vi "TestStepsGui.vi"() -> ()   [LabVIEW 2016]
uses:
  TestStepsGui.Action.ctl
  <vilib>/Utility/miscctls.llb/LVRowAndColumnUnsignedTypeDef.ctl
  <vilib>/Utility/miscctls.llb/LVRowAndColumnTypeDef.ctl
  tools/CitTemplate/citTemplate.errData.ctl
  tools/EventLog/EventLog.EventSource.ctl
  Sequence/Sequence.Data.ctl
  Sequence/Sequence.State.ctl
  Sequence/Sequence.Step.Status.ctl
  Sequence/Sequence.Test.BreakReason.ctl
  Sequence/Sequence.Test.BreakSource.ctl
  Sequence/Sequence.Test.Status.ctl
  Sequence/Sequence.Slot.StatusData.ctl
  Sequence/Sequence.Test.Unload.Status.ctl
  Sequence/Sequence.Prod.StatusData.ctl
  Sequence/Sequence.UserActions.ctl
  Sequence/Sequence.UserData.ctl
  Sequence/Sequence.MainMode.ctl
  MainGui.TestOptions.ctl
  Sequence/Sequence.Code.Sets.ctl
  Sequence/Sequence.PlateType.ctl
  Logger/Logger.Variant.Sets.ctl
  Station/Station.Changeover.State.vi
  Station/Station.Plate.Properties.ctl
  Sequence/Sequence.Code.SerialFormat.ctl
  Drivers/V7310/LowLevel/V7310.Job.Sets.ctl
  Sequence/Sequence.Counters.ctl
  Sequence/Sequence.Global.vi
  Global/ApplicationGlobal.vi
panel:
  out "Part":string
  out "Prog":bool
  out "ClientPlate":picture
  out "Total":u16 caption="Wymagane"
  out "NOK":u16
  out "OK":u16
  out "Done":u16 caption="Zrobione"
  out "Image B":picture caption="B - 0 - ERROR - 0 %"
  out "Image A":picture caption="A - 0 - ERROR - 0 %"
  out "_loop":i32(ring)=4
  out "Started":bool
  out "Panel":refnum<vi>
  in  "StartHere...":bool
  in  "LastCodes":i32(listbox) caption="Last A"
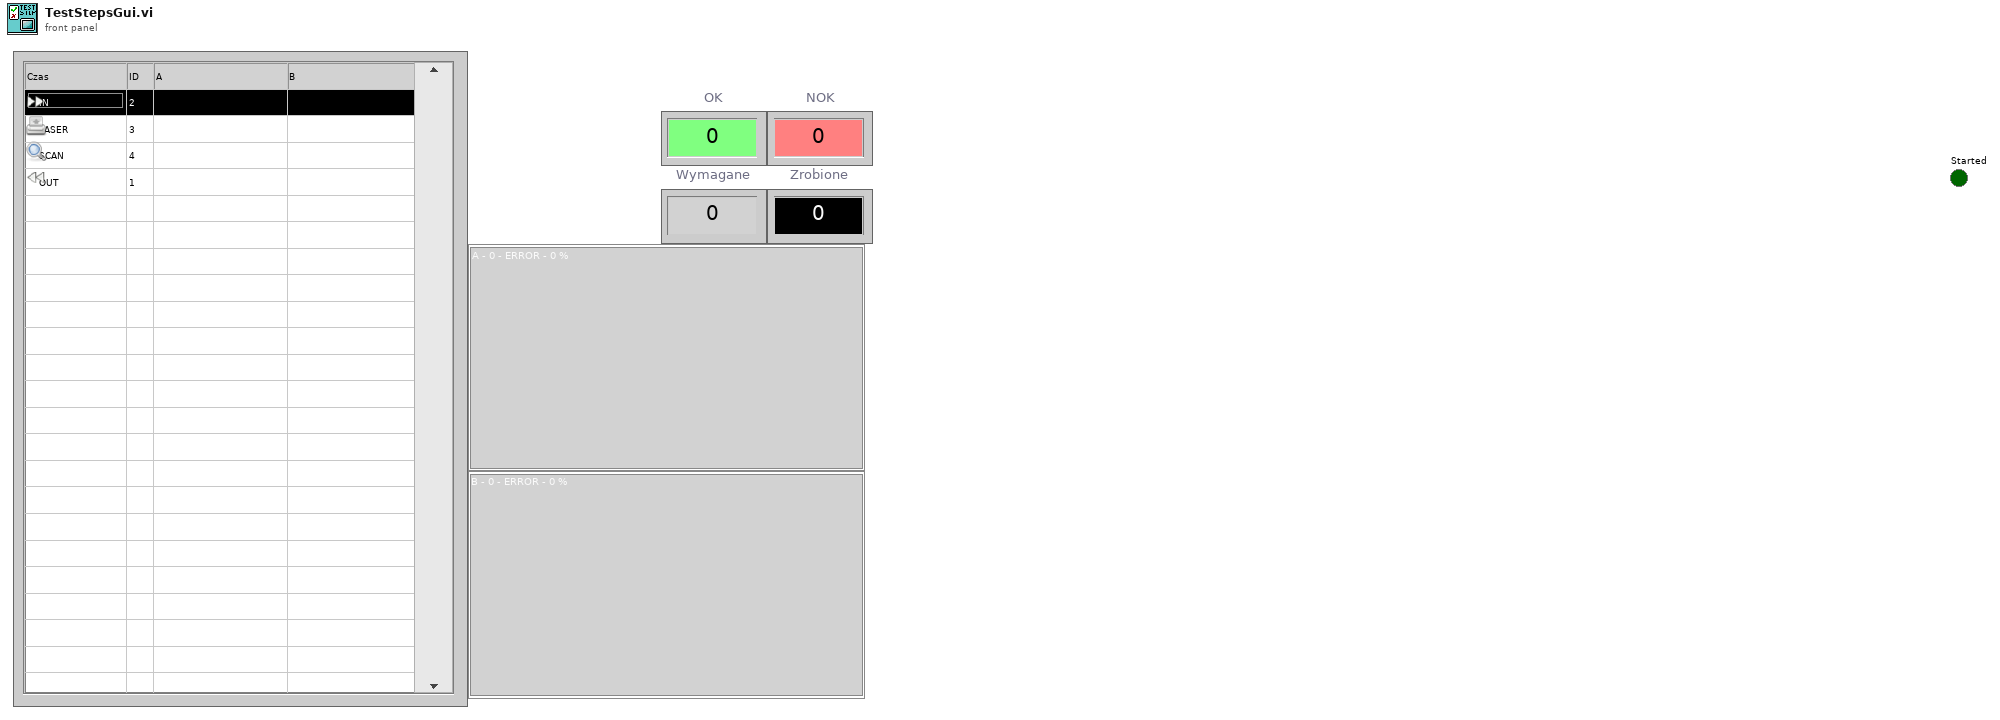
[diagram p1: front panel]
types:
  T1 = typedef "TestStepsGui.Action.ctl" = enum32{"idle", "constructor", "destructor", "--- TestStepsGui ---", "Select", "Load", "Start", "Update", "Update Images"}
  T2 = typedef "LVRowAndColumnTypeDef.ctl" = cluster{"Row":i32, "Column":i32}
  T3 = typedef "LVRowAndColumnUnsignedTypeDef.ctl" = cluster{"Row":u32, "Column":u32}
  T4 = typedef "citTemplate.errData.ctl" = cluster{"ts":timestamp, "src":T5, "instance":i32, "action":string, "error":errorcluster, "unconfirmed":bool}
  T5 = typedef "EventLog.EventSource.ctl" = enum16{"All", "Gui", "Ref", "File", "Arch", "Seq", "CPX", "DB", "Laser", "Scan.P", "Scan.O"}
  T6 = typedef "Sequence.Data.ctl" = cluster{"BeginTS":timestamp, "EndTS":timestamp, "State":T7, "Status.Work":T8, "Status.Process":T8, "Status.Home":T8, "Status.Wabco":T8, "Status.Client":T8, "BreakReason":T9, "BreakSource":T10, "DoorLock":bool, "Status.Prod":T11[], "UserAction":T15, "UserData":T16, "Error":errorcluster, "Code":T19, "Rotations":i32, "ProdIdx":i32, "ProdDone":T11[], "PrintedSerials-Wabco":i32[], "PrintedSerials-Client":i32[], "Counters-Wabco":T26, "Counters-Client":T26}
  T7 = typedef "Sequence.State.ctl" = enum16{"Init", "Idle", "Home", "Work", "Run", "Pause"}
  T8 = typedef "Sequence.Step.Status.ctl" = enum16{"-", "Pending", "Running", "Skipped", "Passed", "Failed", "Done", "Error", "Aborted", "Stopped"}
  T9 = typedef "Sequence.Test.BreakReason.ctl" = enum16{"-", "NOK container", "OK container", "Rev empty", "Rev missing", "Rev wrong", "Fork missing", "Fork wrong", "NOK limit", "Unload failure", "Single slot", "Part done", "Err: Prod move work", "Err: Prod move home", "Err: Prod lift work", "Err: Prod lift home", "Err: Prod Arm Work", "Err: Prod Arm NOK", "Err: Prod Arm OK", "Err: Prod NOK suck", "Err: Prod NOK drop", "Err: Prod OK missing", "Err: Prod OK suck", "Err: Prod OK drop"}
  T10 = typedef "Sequence.Test.BreakSource.ctl" = enum16{"-", "A", "B", "A/B"}
  T11 = typedef "Sequence.Test.Status.ctl" = cluster{"Slot":T12, "A":T14, "B":T14}
  T12 = typedef "Sequence.Slot.StatusData.ctl" = cluster{"ID":i32, "Unload":T13, "TS":timestamp, "duration":u32}
  T13 = typedef "Sequence.Test.Unload.Status.ctl" = enum16{"init", "check NOK", "check OK", "wait on NOK", "wait on OK", "wait on Unload", "done"}
  T14 = typedef "Sequence.Prod.StatusData.ctl" = cluster{"status":T8, "pause":T9, "present":bool, "printed":bool, "scanned":bool, "tuned":bool, "removed":bool, "serial":i32, "code":string, "path":path, "corners":cluster{"X":i32, "Y":i32}[], "verification":u8}
  T15 = typedef "Sequence.UserActions.ctl" = cluster{"Stop":bool, "Pause":bool, "Next":bool}
  T16 = typedef "Sequence.UserData.ctl" = cluster{"GuiMode":T17, "Test":T18, "ContinueOrder":bool}
  T17 = typedef "Sequence.MainMode.ctl" = enum16{"Process", "Base", "Order", "Manual", "Logs", "Results", "Stats", "DMC Config"}
  T18 = typedef "MainGui.TestOptions.ctl" = cluster{"IgnoreResults":bool, "IgnoreImages":bool, "ServiceMode":bool}
  T19 = typedef "Sequence.Code.Sets.ctl" = cluster{"Ready":bool, "DoubleOrder":bool, "OrderDone":bool, "AllowSingleSlot":bool, "TunedA":bool, "TunedB":bool, "CheckDM":bool, "ThresholdA":u8, "ThresholdB":u8, "Plate":T20, "ImgPath":path, "Variant":T21}
  T20 = typedef "Sequence.PlateType.ctl" = enum16{"Wabco", "Client"}
  T21 = typedef "Logger.Variant.Sets.ctl" = cluster{"State":T22, "ImgPath":path, "WabcoPlate":string, "WabcoProduct":string, "ClientProduct":string, "ClientPlate":string, "TotalQuantity":u16, "OrderQuantity":u16, "Serial":i32, "Wabco":T23, "Client":T23}
  T22 = typedef "Station.Changeover.State.vi" = enum16{"Init", "Scaning", "NOK", "Wait for ack", "Ready"}
  T23 = typedef "Station.Plate.Properties.ctl" = cluster{"LaserJob":string, "AdditionalTxt":string, "FactoryCode":string, "RevID":u8, "ForkID":u8, "FailuresLimit":u16, "GlobalCnt":i32, "Bank":u8, "SerialFormat":T24, "CoordA":T25, "CoordB":T25, "DMCconfig":i32}
  T24 = typedef "Sequence.Code.SerialFormat.ctl" = enum8{"", "6 dig", "7 dig"}
  T25 = typedef "V7310.Job.Sets.ctl" = cluster{"X":dbl, "Y":dbl, "Angle":dbl}
  T26 = typedef "Sequence.Counters.ctl" = cluster{"Expected":u16, "Done":u16, "OK":u16, "NOK":u16, "NOKlimit":u16, "Part":u16, "PartOK":u16}
  T27 = typedef "citTemplate.notifierHandle.ctl" = refnum<notifier>
  T28 = enum32{"Invalid", "Standard", "Closed", "Hidden", "Minimized", "Maximized"}
  T29 = typedef "LVPositionTypeDef.ctl" = cluster{"Left":i32, "Top":i32}
  T30 = typedef "imagedata.ctl" = cluster{"image type":i32, "image depth":i32, "image":u8[], "mask":u8[], "colors":u32[], "Rectangle":cluster{"left":i16, "top":i16, "right":i16, "bottom":i16}}
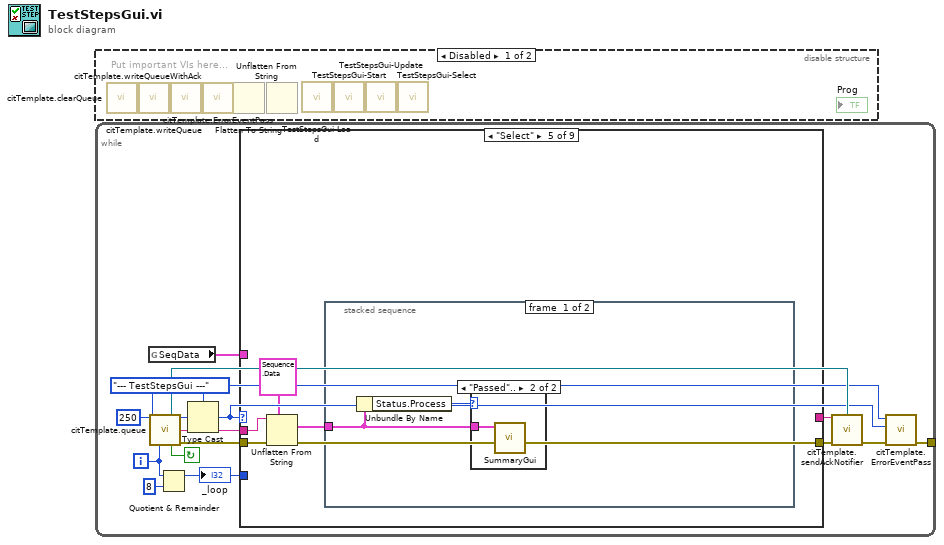
[diagram p0: block diagram]
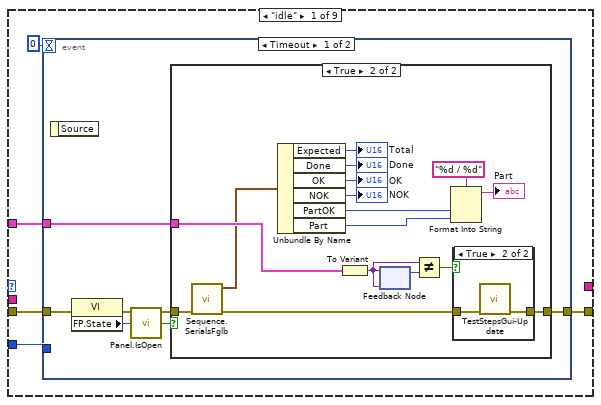
[diagram p3: hidden frame]
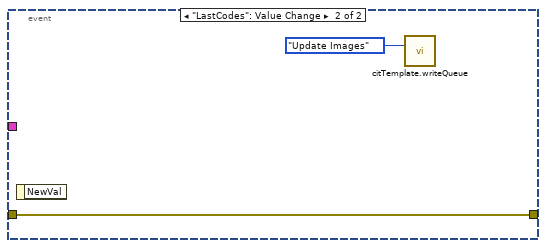
[diagram p6: hidden frame]
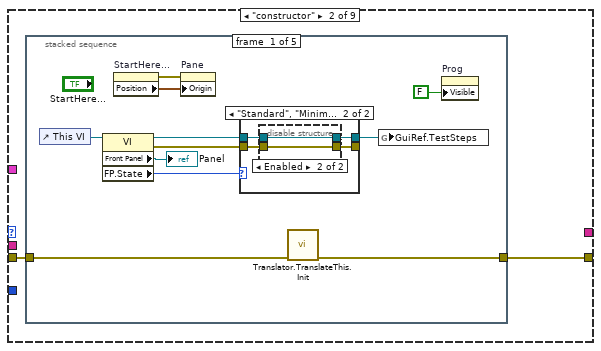
[diagram p7: hidden frame]
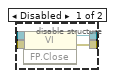
[diagram p9: hidden frame]
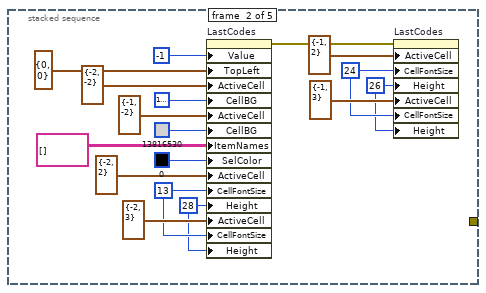
[diagram p10: hidden frame]
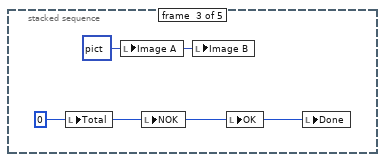
[diagram p11: hidden frame]
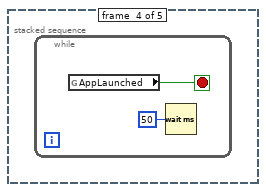
[diagram p12: hidden frame]
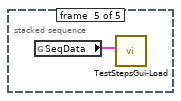
[diagram p13: hidden frame]
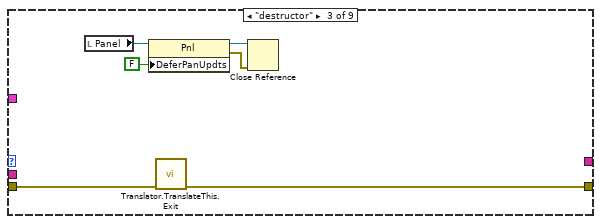
[diagram p14: hidden frame]
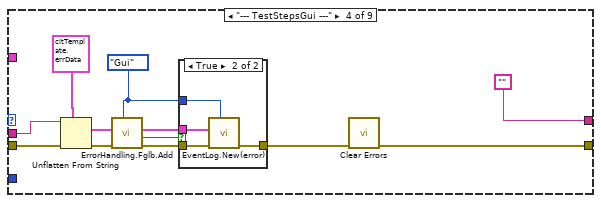
[diagram p15: hidden frame]
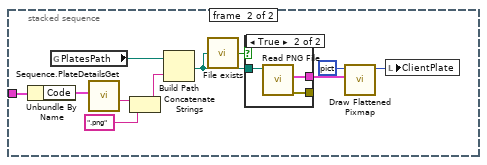
[diagram p18: hidden frame]
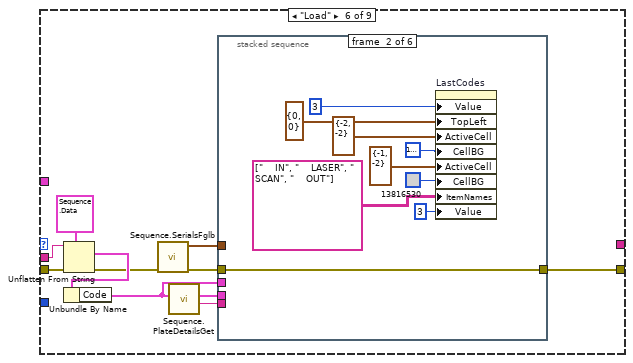
[diagram p20: hidden frame]
diagram:
  n1 = disable-structure shown="Disabled" {
    frame Disabled {
      # "Put important VIs here..."
      n2 = call "citTemplate.clearQueue.vi"() -> ()  [unwired: 14 in, 2 out]
      n3 = call "citTemplate.writeQueue.vi"() -> ()  [unwired: 15 in, 1 out]
      n4 = call "citTemplate.writeQueueWithAck.vi"() -> ()  [unwired: 13 in, 3 out]
      n5 = call "citTemplate.ErrorEventPass.vi"() -> ()  [unwired: 11 in, 1 out]
      n6 = Flatten To String() -> ()  [unwired: 4 in, 3 out]
      n7 = Unflatten From String() -> ()  [unwired: 5 in, 3 out]
      n8 = call "TestStepsGui-Load.vi"() -> ()  [unwired: 11 in, 1 out]
      n9 = call "TestStepsGui-Start.vi"() -> ()  [unwired: 11 in, 1 out]
      n10 = call "TestStepsGui-Update.vi"() -> ()  [unwired: 11 in, 1 out]
      n11 = call "TestStepsGui-Select.vi"() -> ()  [unwired: 11 in, 1 out]
    }
    frame Enabled {
    }
  }
  n12 = while {
    tunnel: [w4] -> _
    i -> [w6]
    stop <- w12 continue-if-true
    w9 = TestStepsGui.Action."--- TestStepsGui ---" ("Action")
    n13 = global read "Sequence.Global.vi" "SeqData"() -> (w1:T6)
    n14 = call "citTemplate.queue.vi"("ms timeout (250 ms)"=250, "event enum"=w9, "iteration (-1)"=w6) -> ("notifierHandle out"=w11:T27, "event out"=w15:u32, "(flatten) data out"=w14:string, "continue"=w12:bool, "error out"=w13:errorcluster)  [unwired: 2 in, 6 out]
    n15 = Quotient & Remainder(x=w6, y=8) -> (x-y*floor(x/y)=w2:i32)  [unwired: 1 out]
    "_loop" <- w2
    n16 = Type Cast(type=w9, x=w15) -> (*(type *) &x=w5:T1)
    n17 = case shown="\"Select\"" w5 {
      tunnel: w14 -> [_ _ _ w111 w121 w148 w204 _ _]
      tunnel: w13 -> [w19 w50 w100 w110 w122 w150 w205 w207 w267]
      tunnel: [_ _ _ "" _ _ _ _ _] -> w10
      tunnel: [w18 w49 w101 w103 w120 w149 w199 w208 w267] -> w8
      tunnel: w2 -> [w17 _ _ _ _ _ _ _ _]
      tunnel: w1 -> [w16 _ _ _ _ _ _ w206 w259]
      frame "idle" {
        n18 = event shown="[0] Timeout" {
          selector: _ -> [_ _]
          dyn-events: _ -> [_ _]
          timeout: 0 -> [_ _]
          tunnel: w19 -> [w26 w48]
          tunnel: [w25 w48] -> w18
          tunnel: w17 -> [_ _]
          tunnel: w16 -> [w23 _]
          event Timeout {
            n19 = event-data() -> ()  [unwired: 1 in, 1 out]
            n20 = property class="VI"(error in=w26) -> (error out=w24:errorcluster, "FP.State"=w22:T28)  [unwired: 1 in, 1 out]
            n21 = call "Panel.IsOpen.vi"("FP State"=w22) -> ("Open?"=w21:bool)
            n22 = case shown="True" w21 {
              tunnel: w24 -> [w27 w34]
              tunnel: [w27 w43] -> w25
              tunnel: w23 -> [_ w35]
              frame False {
              }
              frame True {
                n23 = call "Sequence.SerialsFglb.vi"("error in"=w34) -> ("error out"=w33:errorcluster, "Counters out"=w29:T26)  [unwired: 6 in, 3 out]
                n24 = Unbundle By Name(w29) -> ("Expected"=→"Total":u16, "Done"=→"Done":u16, "OK"=→"OK":u16, "NOK"=→"NOK":u16, "PartOK"=w32:u16, "Part"=w28:u16)
                n25 = To Variant(anything=w35) -> (Variant=w41:variant)
                n26 = feedback #1(w41) -> (w42:variant)
                n27 = feedback-in #1(w41) -> ()
                n28 = Not Equal?(x=w41, y=w42) -> (x != y?=w36:bool)
                n29 = Format Into String(format string="%d / %d", w32, w28) -> (resulting string=→"Part":string)  [unwired: 2 in, 1 out]
                n30 = case shown="True" w36 {
                  tunnel: w33 -> [w44 w45]
                  tunnel: [w44 w46] -> w43
                  frame False {
                  }
                  frame True {
                    n31 = call "TestStepsGui-Update.vi"("error in"=w45) -> ("error out"=w46:errorcluster)  [unwired: 10 in]
                  }
                }
              }
            }
          }
          event "LastCodes": Value Change {
            n32 = event-data() -> ()  [unwired: 1 in, 1 out]
            n33 = call "citTemplate.writeQueue.vi"("event in (if not connected:all statemachine with data event)"=TestStepsGui.Action."Update Images" ("Action")) -> ()  [unwired: 14 in, 1 out]
          }
        }
      }
      frame "constructor" {
        n34 = stacked-sequence {
          tunnel: w50 -> [w57 _ _ _ _]
          tunnel: [w52 _ _ _ _] -> w49
          frame #0 {
            n35 = control-ref of="This VI"() -> (w58:refnum<vi>)
            n36 = property class="VI"(reference=w58) -> (reference out=w56:refnum<vi>, error out=w55:errorcluster, "Front Panel"=→"Panel":refnum<vi>, "FP.State"=w54:T28)  [unwired: 1 in]
            n37 = property on="StartHere..." class="Bool (strict)"() -> (error out=w60:errorcluster, "Position"=w59:T29)  [unwired: 2 in, 1 out]
            n38 = property on="Pane" class="Pane"(error in=w60, "Origin"=w59) -> ()  [unwired: 1 in, 2 out]
            n39 = case shown="\"Standard\", \"Minimized\", \"Maximized\"" w54 {
              tunnel: w56 -> [w63 w67]
              tunnel: w55 -> [w62 w66]
              tunnel: [w63 w65] -> w53
              tunnel: [w62 w64] -> _
              frame Default {
              }
              frame "Standard", "Minimized", "Maximized" {
                n40 = disable-structure shown="Enabled" {
                  disable-tunnel: w67 -> [w71 w73]
                  disable-tunnel: w66 -> [w70 w72]
                  disable-tunnel: [w69 w73] -> w65
                  disable-tunnel: [w68 w72] -> w64
                  frame Disabled {
                    n41 = invoke class="VI" method="FP.Close"(reference=w71, error in=w70) -> (reference out=w69:refnum<vi>, error out=w68:errorcluster)  [unwired: 1 in, 1 out]
                  }
                  frame Enabled {
                  }
                }
              }
            }
            n42 = call "Translator.TranslateThis.Init.vi"("error in"=w57) -> ("error out"=w52:errorcluster)  [unwired: 10 in]
            n43 = global write "ApplicationGlobal.vi" "GuiRef.TestSteps"(w53) -> ()
            n44 = property on="Prog" class="Bool (strict)"("Visible"=FALSE) -> ()  [unwired: 2 in, 2 out]
          }
          frame #1 {
            w75 = u32 26 ("Active Cell:Cell Size:Height")
            w76 = u32 24 ("Active Cell:Cell Font:Size")
            w79 = u32 28 ("Active Cell:Cell Size:Height")
            w80 = u32 13 ("Active Cell:Cell Font:Size")
            n45 = property on="LastCodes" class="MCListbox (strict)"("Value"=-1 ("Last A"), "TopLeft"=T3 {"Row"=0, "Column"=0} ("Top Left Visible Cell"), "ActiveCell"=T2 {"Row"=-2, "Column"=-2} ("Active Cell:Active Cell"), "CellBG"=u32 16777226, "ActiveCell"=T2 {"Row"=-1, "Column"=-2} ("Active Cell:Active Cell"), "CellBG"=u32 13816530, "ItemNames"=string[][] [] ("Item Names"), "SelColor"=u32 0, "ActiveCell"=T2 {"Row"=-2, "Column"=2} ("Active Cell:Active Cell"), "CellFontSize"=w80, "Height"=w79, "ActiveCell"=T2 {"Row"=-2, "Column"=3} ("Active Cell:Active Cell"), "CellFontSize"=w80, "Height"=w79) -> (error out=w74:errorcluster)  [unwired: 2 in, 1 out]
            n46 = property on="LastCodes" class="MCListbox (strict)"(error in=w74, "ActiveCell"=T2 {"Row"=-1, "Column"=2} ("Active Cell:Active Cell"), "CellFontSize"=w76, "Height"=w75, "ActiveCell"=T2 {"Row"=-1, "Column"=3} ("Active Cell:Active Cell"), "CellFontSize"=w76, "Height"=w75) -> ()  [unwired: 1 in, 2 out]
          }
          frame #2 {
            w91 = u16 0 ("Expected")
            w92 = picture data[5B] ("Image A")
            n47 = local write "Total"(w91) -> ()
            n48 = local write "Image A"(w92) -> ()
            n49 = local write "NOK"(w91) -> ()
            n50 = local write "Image B"(w92) -> ()
            n51 = local write "OK"(w91) -> ()
            n52 = local write "Done"(w91) -> ()
          }
          frame #3 {
            n53 = while {
              stop <- w94 stop-if-true
              n54 = global read "ApplicationGlobal.vi" "AppLaunched"() -> (w94:bool)
              n55 = Wait (ms)(milliseconds to wait=u32 50) -> ()  [unwired: 1 out]
            }
          }
          frame #4 {
            n56 = global read "Sequence.Global.vi" "SeqData"() -> (w95:T6)
            n57 = call "TestStepsGui-Load.vi"("Data"=w95) -> ()  [unwired: 10 in, 1 out]
          }
        }
      }
      frame "destructor" {
        n58 = local read "Panel"() -> (w97:refnum<vi>)
        n59 = property class="Pnl"(reference=w97, "DeferPanUpdts"=FALSE ("Defer Panel Updates")) -> (reference out=w99:refnum<vi>, error out=w96:errorcluster)  [unwired: 1 in]
        n60 = call "Translator.TranslateThis.Exit.vi"("error in"=w100) -> ("error out"=w101:errorcluster)  [unwired: 10 in]
        n61 = Close Reference(reference=w99, error in (no error)=w96) -> ()  [unwired: 1 out]
      }
      frame "--- TestStepsGui ---" {
        w106 = EventLog.EventSource."Gui" ("Event source")
        n62 = Unflatten From String(type=T4 {"ts"=timestamp(0 s since 1904-01-01), "src"=enum."All", "instance"=0, "action"="", "error"={"status"=FALSE, "code"=0, "source"=""}, "unconfirmed"=FALSE} ("ErrData"), binary string=w111, error in (no error)=w110) -> (value=w102:T4, error out=w104:errorcluster)  [unwired: 3 out]
        n63 = call "ErrorHandling.Fglb.Add.vi"("Event source"=w106, "error in (no error)"=w104, "Error in"=w102) -> ("error out"=w108:errorcluster, "changed?"=w107:bool)  [unwired: 7 in]
        n64 = case shown="True" w107 {
          tunnel: [w113 w117] -> w105
          tunnel: w102 -> [_ w116]
          tunnel: w108 -> [w113 w115]
          tunnel: w106 -> [_ w114]
          frame False {
          }
          frame True {
            n65 = call "EventLog.New(error).vi"("Source (All)"=w114, "error in"=w115, "ErrData"=w116) -> ("error out"=w117:errorcluster)  [unwired: 8 in]
          }
        }
        n66 = call <vilib>:"Clear Errors.vi"("error in (no error)"=w105) -> ("error out"=w103:errorcluster)  [unwired: 5 in, 1 out]
      }
      frame "Select" {
        n67 = Unflatten From String(type=T6 {"BeginTS"=timestamp(0 s since 1904-01-01), "EndTS"=timestamp(0 s since 1904-01-01), "State"=enum."Init", "Status.Work"=enum."-", "Status.Process"=enum."-", "Status.Home"=enum."-", "Status.Wabco"=enum."-", "Status.Client"=enum."-", "BreakReason"=enum."-", "BreakSource"=enum."-", "DoorLock"=FALSE, "Status.Prod"=[], "UserAction"={"Stop"=FALSE, "Pause"=FALSE, "Next"=FALSE}, "UserData"={"GuiMode"=enum."Process", "Test"={"IgnoreResults"=FALSE, "IgnoreImages"=FALSE, "ServiceMode"=FALSE}, "ContinueOrder"=FALSE}, "Error"={"status"=FALSE, "code"=0, "source"=""}, "Code"={"Ready"=FALSE, "DoubleOrder"=FALSE, "OrderDone"=FALSE, "AllowSingleSlot"=FALSE, "TunedA"=FALSE, "TunedB"=FALSE, "CheckDM"=FALSE, "ThresholdA"=0, "ThresholdB"=0, "Plate"=enum."Wabco", "ImgPath"=path "", "Variant"={"State"=enum."Init", "ImgPath"=path "", "WabcoPlate"="", "WabcoProduct"="", "ClientProduct"="", "ClientPlate"="", "TotalQuantity"=0, "OrderQuantity"=0, "Serial"=0, "Wabco"={"LaserJob"="", "AdditionalTxt"="", "FactoryCode"="", "RevID"=0, "ForkID"=0, "FailuresLimit"=0, "GlobalCnt"=0, "Bank"=0, "SerialFormat"=enum."", "CoordA"={"X"=0.0, "Y"=0.0, "Angle"=0.0}, "CoordB"={"X"=0.0, "Y"=0.0, "Angle"=0.0}, "DMCconfig"=0}, "Client"={"LaserJob"="", "AdditionalTxt"="", "FactoryCode"="", "RevID"=0, "ForkID"=0, "FailuresLimit"=0, "GlobalCnt"=0, "Bank"=0, "SerialFormat"=enum."", "CoordA"={"X"=0.0, "Y"=0.0, "Angle"=0.0}, "CoordB"={"X"=0.0, "Y"=0.0, "Angle"=0.0}, "DMCconfig"=0}}}, "Rotations"=0, "ProdIdx"=0, "ProdDone"=[], "PrintedSerials-Wabco"=[], "PrintedSerials-Client"=[], "Counters-Wabco"={"Expected"=0, "Done"=0, "OK"=0, "NOK"=0, "NOKlimit"=0, "Part"=0, "PartOK"=0}, "Counters-Client"={"Expected"=0, "Done"=0, "OK"=0, "NOK"=0, "NOKlimit"=0, "Part"=0, "PartOK"=0}} ("Data"), binary string=w121, error in (no error)=w122) -> (value=w118:T6, error out=w120:errorcluster)  [unwired: 3 out]
        n68 = stacked-sequence {
          tunnel: w118 -> [w123 w126]
          frame #0 {
            n69 = Unbundle By Name(w123) -> ("Status.Process"=w124:T8)
            n70 = case shown="\"Passed\".." w124 {
              tunnel: w123 -> [_ w125]
              frame "-", Default {
              }
              frame "Passed".. {
                n71 = call "SummaryGui.vi"("SeqData"=w125) -> ()  [unwired: 11 in]
              }
            }
          }
          frame #1 {
            n72 = Unbundle By Name(w126) -> ("Code"=w129:T19)
            n73 = global read "ApplicationGlobal.vi" "PlatesPath"() -> (w127:path)
            n74 = call "Sequence.PlateDetailsGet.vi"("Code in"=w129) -> ("PlateNo"=w136:string)  [unwired: 9 in, 1 out]
            n75 = Concatenate Strings(w136, ".png" ("string")) -> (w130:string)
            n76 = Build Path(base path=w127, name or relative path=w130) -> (appended path=w134:path)
            n77 = call "File exists.vi"("file path"=w134) -> ("exists?"=w131:bool)  [unwired: 4 in]
            n78 = case shown="True" w131 {
              tunnel: w134 -> [_ w139]
              tunnel: [_ w138] -> w133
              tunnel: [_ w137] -> _
              frame False {
              }
              frame True {
                n79 = call <vilib>:"Read PNG File.vi"("path to PNG file"=w139) -> ("error out"=w137:errorcluster, "image data"=w138:T30)  [unwired: 8 in, 1 out]
              }
            }
            n80 = call <vilib>:"Draw Flattened Pixmap.vi"("image data"=w133, "picture"=picture data[5B]) -> ("new picture"=w135:picture)  [unwired: 7 in]
            n81 = local write "ClientPlate"(w135) -> ()
          }
        }
      }
      frame "Load" {
        n82 = Unflatten From String(type=T6 {"BeginTS"=timestamp(0 s since 1904-01-01), "EndTS"=timestamp(0 s since 1904-01-01), "State"=enum."Init", "Status.Work"=enum."-", "Status.Process"=enum."-", "Status.Home"=enum."-", "Status.Wabco"=enum."-", "Status.Client"=enum."-", "BreakReason"=enum."-", "BreakSource"=enum."-", "DoorLock"=FALSE, "Status.Prod"=[], "UserAction"={"Stop"=FALSE, "Pause"=FALSE, "Next"=FALSE}, "UserData"={"GuiMode"=enum."Process", "Test"={"IgnoreResults"=FALSE, "IgnoreImages"=FALSE, "ServiceMode"=FALSE}, "ContinueOrder"=FALSE}, "Error"={"status"=FALSE, "code"=0, "source"=""}, "Code"={"Ready"=FALSE, "DoubleOrder"=FALSE, "OrderDone"=FALSE, "AllowSingleSlot"=FALSE, "TunedA"=FALSE, "TunedB"=FALSE, "CheckDM"=FALSE, "ThresholdA"=0, "ThresholdB"=0, "Plate"=enum."Wabco", "ImgPath"=path "", "Variant"={"State"=enum."Init", "ImgPath"=path "", "WabcoPlate"="", "WabcoProduct"="", "ClientProduct"="", "ClientPlate"="", "TotalQuantity"=0, "OrderQuantity"=0, "Serial"=0, "Wabco"={"LaserJob"="", "AdditionalTxt"="", "FactoryCode"="", "RevID"=0, "ForkID"=0, "FailuresLimit"=0, "GlobalCnt"=0, "Bank"=0, "SerialFormat"=enum."", "CoordA"={"X"=0.0, "Y"=0.0, "Angle"=0.0}, "CoordB"={"X"=0.0, "Y"=0.0, "Angle"=0.0}, "DMCconfig"=0}, "Client"={"LaserJob"="", "AdditionalTxt"="", "FactoryCode"="", "RevID"=0, "ForkID"=0, "FailuresLimit"=0, "GlobalCnt"=0, "Bank"=0, "SerialFormat"=enum."", "CoordA"={"X"=0.0, "Y"=0.0, "Angle"=0.0}, "CoordB"={"X"=0.0, "Y"=0.0, "Angle"=0.0}, "DMCconfig"=0}}}, "Rotations"=0, "ProdIdx"=0, "ProdDone"=[], "PrintedSerials-Wabco"=[], "PrintedSerials-Client"=[], "Counters-Wabco"={"Expected"=0, "Done"=0, "OK"=0, "NOK"=0, "NOKlimit"=0, "Part"=0, "PartOK"=0}, "Counters-Client"={"Expected"=0, "Done"=0, "OK"=0, "NOK"=0, "NOKlimit"=0, "Part"=0, "PartOK"=0}} ("Data"), binary string=w148, error in (no error)=w150) -> (value=w146:T6, error out=w143:errorcluster)  [unwired: 2 in, 1 out]
        n83 = Unbundle By Name(w146) -> ("Code"=w140:T19)
        n84 = call "Sequence.SerialsFglb.vi"("error in"=w143) -> ("error out"=w142:errorcluster, "Counters out"=w141:T26)  [unwired: 6 in, 3 out]
        n85 = call "Sequence.PlateDetailsGet.vi"("Code in"=w140) -> ("PlateNo"=w144:string, "PlateDetails"=w145:T23)  [unwired: 9 in]
        n86 = stacked-sequence {
          tunnel: w142 -> [_ w161 _ _ _ _]
          tunnel: [_ w161 _ _ _ _] -> w149
          tunnel: w145 -> [_ _ _ _ _ _]
          tunnel: w144 -> [_ _ w163 _ _ _]
          tunnel: w141 -> [_ _ _ _ w195 _]
          tunnel: w140 -> [_ _ _ w175 _ _]
          frame #0 {
            n87 = local read "Panel"() -> (w151:refnum<vi>)
            n88 = property class="Pnl"(reference=w151, "DeferPanUpdts"=TRUE ("Defer Panel Updates")) -> ()  [unwired: 1 in, 2 out]
          }
          frame #1 {
            n89 = property on="LastCodes" class="MCListbox (strict)"("Value"=3 ("Last A"), "TopLeft"=T3 {"Row"=0, "Column"=0} ("Top Left Visible Cell"), "ActiveCell"=T2 {"Row"=-2, "Column"=-2} ("Active Cell:Active Cell"), "CellBG"=u32 16777226, "ActiveCell"=T2 {"Row"=-1, "Column"=-2} ("Active Cell:Active Cell"), "CellBG"=u32 13816530, "ItemNames"=string[][] [["    IN"], ["    LASER"], ["    SCAN"], ["    OUT"]] ("Item Names"), "Value"=3 ("LastCodes")) -> ()  [unwired: 2 in, 2 out]
          }
          frame #2 {
            n90 = global read "ApplicationGlobal.vi" "PlatesPath"() -> (w169:path)
            n91 = Concatenate Strings(w163, ".png" ("string")) -> (w170:string)
            n92 = Build Path(base path=w169, name or relative path=w170) -> (appended path=w164:path)
            n93 = call "File exists.vi"("file path"=w164) -> ("exists?"=w168:bool)  [unwired: 4 in]
            n94 = case shown="True" w168 {
              tunnel: w164 -> [_ w174]
              tunnel: [_ w173] -> w166
              tunnel: [_ w172] -> _
              frame False {
              }
              frame True {
                n95 = call <vilib>:"Read PNG File.vi"("path to PNG file"=w174) -> ("error out"=w172:errorcluster, "image data"=w173:T30)  [unwired: 8 in, 1 out]
              }
            }
            n96 = call <vilib>:"Draw Flattened Pixmap.vi"("image data"=w166, "picture"=picture data[5B]) -> ("new picture"=→"ClientPlate":picture)  [unwired: 7 in]
            n97 = property on="Prog" class="Bool (strict)"("Visible"=FALSE) -> ()  [unwired: 2 in, 2 out]
          }
          frame #3 {
            n98 = Unbundle By Name(w175) -> ("CheckDM"=w176:bool)
            n99 = case shown="True" w176 {
              tunnel: [u32 24 ("Active Cell:Cell Font:Size") u32 24 ("Active Cell:Cell Font:Size")] -> w181
              tunnel: [u32 26 ("Active Cell:Cell Size:Height") u32 26 ("Active Cell:Cell Size:Height")] -> w182
              tunnel: [u32 26 ("Active Cell:Cell Size:Height") u32 26 ("Active Cell:Cell Size:Height")] -> w177
              tunnel: [u32 24 ("Active Cell:Cell Font:Size") u32 13 ("Active Cell:Cell Font:Size")] -> w178
              frame False {
              }
              frame True {
              }
            }
            n100 = property on="LastCodes" class="MCListbox (strict)"("ActiveCell"=T2 {"Row"=-2, "Column"=2} ("Active Cell:Active Cell"), "CellFontSize"=w178, "Height"=w177, "ActiveCell"=T2 {"Row"=-2, "Column"=3} ("Active Cell:Active Cell"), "CellFontSize"=w178, "Height"=w177, "ActiveCell"=T2 {"Row"=-1, "Column"=2} ("Active Cell:Active Cell"), "CellFontSize"=w181, "Height"=w182, "ActiveCell"=T2 {"Row"=-1, "Column"=3} ("Active Cell:Active Cell"), "CellFontSize"=w181, "Height"=w182) -> ()  [unwired: 2 in, 2 out]
          }
          frame #4 {
            w196 = picture data[5B] ("Image A")
            n101 = Unbundle By Name(w195) -> ("Part"=w194:u16)
            n102 = Greater Than 0?(x=w194) -> (x > 0?=w193:bool)
            n103 = local write "Image A"(w196) -> ()
            n104 = property on="Part" class="Str"("Visible"=w193) -> ()  [unwired: 2 in, 2 out]
            n105 = local write "Image B"(w196) -> ()
          }
          frame #5 {
            n106 = local read "Panel"() -> (w197:refnum<vi>)
            n107 = property class="Pnl"(reference=w197, "DeferPanUpdts"=FALSE ("Defer Panel Updates")) -> ()  [unwired: 1 in, 2 out]
          }
        }
      }
      frame "Start" {
        n108 = Unflatten From String(type=T6 {"BeginTS"=timestamp(0 s since 1904-01-01), "EndTS"=timestamp(0 s since 1904-01-01), "State"=enum."Init", "Status.Work"=enum."-", "Status.Process"=enum."-", "Status.Home"=enum."-", "Status.Wabco"=enum."-", "Status.Client"=enum."-", "BreakReason"=enum."-", "BreakSource"=enum."-", "DoorLock"=FALSE, "Status.Prod"=[], "UserAction"={"Stop"=FALSE, "Pause"=FALSE, "Next"=FALSE}, "UserData"={"GuiMode"=enum."Process", "Test"={"IgnoreResults"=FALSE, "IgnoreImages"=FALSE, "ServiceMode"=FALSE}, "ContinueOrder"=FALSE}, "Error"={"status"=FALSE, "code"=0, "source"=""}, "Code"={"Ready"=FALSE, "DoubleOrder"=FALSE, "OrderDone"=FALSE, "AllowSingleSlot"=FALSE, "TunedA"=FALSE, "TunedB"=FALSE, "CheckDM"=FALSE, "ThresholdA"=0, "ThresholdB"=0, "Plate"=enum."Wabco", "ImgPath"=path "", "Variant"={"State"=enum."Init", "ImgPath"=path "", "WabcoPlate"="", "WabcoProduct"="", "ClientProduct"="", "ClientPlate"="", "TotalQuantity"=0, "OrderQuantity"=0, "Serial"=0, "Wabco"={"LaserJob"="", "AdditionalTxt"="", "FactoryCode"="", "RevID"=0, "ForkID"=0, "FailuresLimit"=0, "GlobalCnt"=0, "Bank"=0, "SerialFormat"=enum."", "CoordA"={"X"=0.0, "Y"=0.0, "Angle"=0.0}, "CoordB"={"X"=0.0, "Y"=0.0, "Angle"=0.0}, "DMCconfig"=0}, "Client"={"LaserJob"="", "AdditionalTxt"="", "FactoryCode"="", "RevID"=0, "ForkID"=0, "FailuresLimit"=0, "GlobalCnt"=0, "Bank"=0, "SerialFormat"=enum."", "CoordA"={"X"=0.0, "Y"=0.0, "Angle"=0.0}, "CoordB"={"X"=0.0, "Y"=0.0, "Angle"=0.0}, "DMCconfig"=0}}}, "Rotations"=0, "ProdIdx"=0, "ProdDone"=[], "PrintedSerials-Wabco"=[], "PrintedSerials-Client"=[], "Counters-Wabco"={"Expected"=0, "Done"=0, "OK"=0, "NOK"=0, "NOKlimit"=0, "Part"=0, "PartOK"=0}, "Counters-Client"={"Expected"=0, "Done"=0, "OK"=0, "NOK"=0, "NOKlimit"=0, "Part"=0, "PartOK"=0}} ("Data"), binary string=w204, error in (no error)=w205) -> (value=w200:T6, error out=w203:errorcluster)  [unwired: 2 in, 1 out]
        n109 = call "TestStepsGui-Load.vi"("error in"=w203, "Data"=w200) -> ("error out"=w199:errorcluster)  [unwired: 9 in]
        "Started" <- TRUE ("Started")
      }
      frame "Update" {
        n110 = stacked-sequence {
          tunnel: [_ w222 _ _] -> w208
          tunnel: w207 -> [_ w219 _ _]
          tunnel: w206 -> [_ w220 w226 _]
          frame #0 {
            n111 = local read "Panel"() -> (w209:refnum<vi>)
            n112 = property class="Pnl"(reference=w209, "DeferPanUpdts"=TRUE ("Defer Panel Updates")) -> ()  [unwired: 1 in, 2 out]
          }
          frame #1 {
            n113 = control-ref of="LastCodes"() -> (w221:refnum<vi>)
            n114 = call "TestStepsGui.Results.Update.vi"("Table"=w221, "error in"=w219, "SeqData"=w220) -> ("error out"=w222:errorcluster, "value out"=w218:T11)  [unwired: 6 in, 1 out]
            n115 = Unbundle By Name(w218) -> ("A.path"=w217:path, "A.corners"=w212:cluster{"X":i32, "Y":i32}[], "B.path"=w215:path, "B.corners"=w213:cluster{"X":i32, "Y":i32}[])
            n116 = call "citTemplate.writeQueue.vi"("event in (if not connected:all statemachine with data event)"=TestStepsGui.Action."Update Images" ("Action")) -> ()  [unwired: 14 in, 1 out]
            n117 = call "Sequence.Prod.LoadImg.vi"("corners"=w212, "path"=w217) -> ("img"=→"Image A":picture)  [unwired: 9 in]
            n118 = call "Sequence.Prod.LoadImg.vi"("corners"=w213, "path"=w215) -> ("img"=→"Image B":picture)  [unwired: 9 in]
          }
          frame #2 {
            n119 = Unbundle By Name(w226) -> ("State"=w225:T7)
            n120 = Greater Or Equal?(x=w225, y=Sequence.State."Run" ("x")) -> (x >= y?=w223:bool)
            n121 = property on="Prog" class="Bool (strict)"("Visible"=w223) -> ()  [unwired: 2 in, 2 out]
          }
          frame #3 {
            n122 = local read "Panel"() -> (w227:refnum<vi>)
            n123 = property class="Pnl"(reference=w227, "DeferPanUpdts"=FALSE ("Defer Panel Updates")) -> ()  [unwired: 1 in, 2 out]
          }
        }
      }
      frame "Update Images" {
        w234 = "%s - %s %%" ("format string")
        n124 = Unbundle By Name(w259) -> ("Status.Prod"=w263:T11[], "ProdDone"=w264:T11[], "ProdIdx"=w261:i32)
        n125 = property on="LastCodes" class="MCListbox (strict)"() -> ("Value"=w260:i32)  [unwired: 2 in, 2 out]
        n126 = Array Subset(array=w264, length=w261) -> (w265:T11[])  [unwired: 1 in]
        n127 = Reverse 1D Array(array=w265) -> (reversed array=w266:T11[])
        n128 = Build Array (concatenate)(w263, w266) -> (w262:T11[])
        n129 = Index Array(array=w262, index=w260) -> (element=w255:T11)
        n130 = Unbundle By Name(w255) -> ("A.serial"=w245:i32, "A.code"=w246:string, "A.path"=w258:path, "A.corners"=w256:cluster{"X":i32, "Y":i32}[], "A.verification"=w233:u8, "B.serial"=w244:i32, "B.code"=w243:string, "B.path"=w257:path, "B.corners"=w240:cluster{"X":i32, "Y":i32}[], "B.verification"=w239:u8)  [unwired: 1 out]
        n131 = call "Sequence.Prod.LoadImg.vi"("corners"=w256, "path"=w258) -> ("img"=w242:picture)  [unwired: 9 in]
        n132 = call "Sequence.Prod.LoadImg.vi"("corners"=w240, "path"=w257) -> ("img"=w241:picture)  [unwired: 9 in]
        n133 = call "Int2Str.vi"("Numeric"=w245) -> ("string"=w253:string)
        n134 = call "Int2Str.vi"("Numeric"=w239) -> ("string"=w237:string)
        n135 = call "Int2Str.vi"("Numeric"=w244) -> ("string"=w248:string)
        n136 = call "Int2Str.vi"("Numeric"=w233) -> ("string"=w232:string)
        n137 = Concatenate Strings(w253, " - " ("string"), w246) -> (w251:string)
        n138 = Concatenate Strings(w248, " - " ("string"), w243) -> (w250:string)
        n139 = Empty String/Path?(string/path=w246) -> (empty?=w254:bool)
        n140 = Select(t=w253, s=w254, f=w251) -> (s? t:f=w231:string)
        n141 = Empty String/Path?(string/path=w243) -> (empty?=w247:bool)
        n142 = Select(t=w248, s=w247, f=w250) -> (s? t:f=w229:string)
        n143 = Format Into String(format string=w234, initial string="A - " ("string"), w231, w232) -> (resulting string=w230:string)  [unwired: 1 in, 1 out]
        n144 = Format Into String(format string=w234, initial string="B - " ("string"), w229, w237) -> (resulting string=w236:string)  [unwired: 1 in, 1 out]
        n145 = property on="Image A" class="Pict"("Caption.Text"=w230, "Value"=w242) -> ()  [unwired: 2 in, 2 out]
        n146 = property on="Image B" class="Pict"("Caption.Text"=w236, "Value"=w241) -> ()  [unwired: 2 in, 2 out]
      }
    }
    n147 = call "citTemplate.sendAckNotifier.vi"("notification data"=w10, "notifierHandle in"=w11, "error in"=w8) -> ()  [unwired: 13 out]
    n148 = call "citTemplate.ErrorEventPass.vi"("error in"=w8, "action of error"=w5, "event in"=w9) -> ("error out"=w4:errorcluster)  [unwired: 2 in, 6 out]
  }
